vi "Reserve Swerve.vi"(7 "Description":string="Reserve", 8 "Command Info":T1, 10 "Command Name":string) -> (0 "Command Info":T1)   [LabVIEW 2023]
uses:
  <vilib>/Rock Robotics/WPI/Framework/Command Status Info.ctl
  <vilib>/Rock Robotics/WPI/Framework/Completion Status.ctl
  <vilib>/Rock Robotics/WPI/Framework/Completion Notifier.ctl
  Implementation/Swerve Setpoints2.ctl
  Implementation/Swerve Operations.ctl
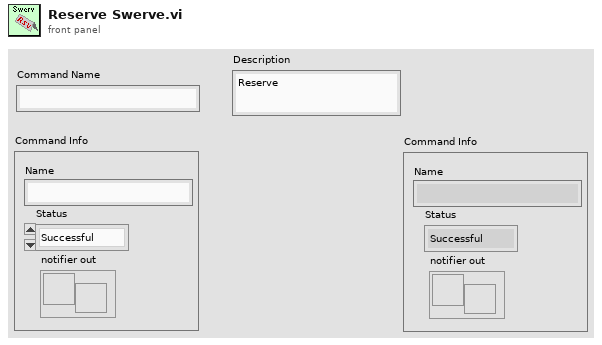
[diagram p1: front panel]
types:
  T1 = typedef "Command Status Info.ctl" = cluster{"Name":string, "Status":T2, "notifier out":T3}
  T2 = typedef "Completion Status.ctl" = enum16{"Successful", "Aborted", "Incomplete"}
  T3 = typedef "Completion Notifier.ctl" = refnum<notifier>
  T4 = typedef "Swerve Setpoints2.ctl" = cluster{"Operation":T5, "Gyro":dbl, "FWD":dbl, "STR":dbl, "X rotate":dbl, "Y rotate":dbl, "Time":dbl, "Distance":dbl, "Right Trigger":dbl, "Angle":dbl, "Start Angle":dbl, "Tag ID":dbl, "Start Positions":dbl[]}
  T5 = typedef "Swerve Operations.ctl" = enum16{"Reserve", "Read Current", "Immediate", "Stop", "Balance", "Direct  Joystick Drive", "Joystick Drive", "Drive for Distance", "Drive for Time", "Turn to Angle", "Drive to Angle(Time)", "Drive to Angle(Distance)", "Look At Cone", "Look At Cube", "Move To Tape", "Move To Tag"}
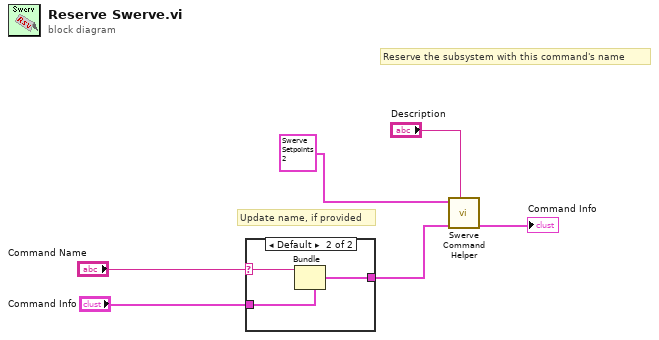
[diagram p0: block diagram]
diagram:
  # "Update name, if provided"
  # "Reserve the subsystem with this command's name"
  n1 = case shown="Default" "Command Name" {
    selector: "Command Name" -> [_ w8]
    tunnel: "Command Info" -> [w7 w10]
    tunnel: [w7 w9] -> w3
    frame "" {
    }
    frame Default {
      n2 = Bundle(cluster=w10, "Name"=w8) -> (w9:T1)  [unwired: 2 in]
    }
  }
  n3 = call "Swerve Command Helper.vi"("Description"="Description", "Command Info In"=w3, "SubSystem Data"=T4 {"Operation"=enum."Reserve", "Gyro"=0.0, "FWD"=0.0, "STR"=0.0, "X rotate"=0.0, "Y rotate"=0.0, "Time"=0.0, "Distance"=0.0, "Right Trigger"=0.0, "Angle"=0.0, "Start Angle"=0.0, "Tag ID"=0.0, "Start Positions"=[]}) -> ("Command Info Out"=→"Command Info":T1)  [unwired: 6 in, 2 out]
